vi "Update Item.vi"(8 "error in (no error)":errorcluster, 9 "Tag":string, 10 "Tree Manager in":refnum<class "Tree Manager.lvclass">, 11 "Data Item in":refnum<class "Data Item.lvclass">) -> (0 "error out":errorcluster, 2 "Tree Manager out":refnum<class "Tree Manager.lvclass">, 3 "Data Item out":refnum<class "Data Item.lvclass">)   [LabVIEW 2026, in "VILab.lvlib" / "Data Item.lvclass"]
uses:
  Data Item.lvclass
  Data Item.lvclass/Data Item.ctl
  Tree Manager/Tree Manager.lvclass
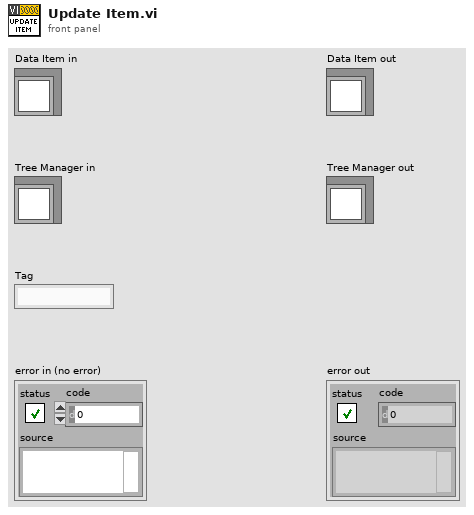
[diagram p1: front panel]
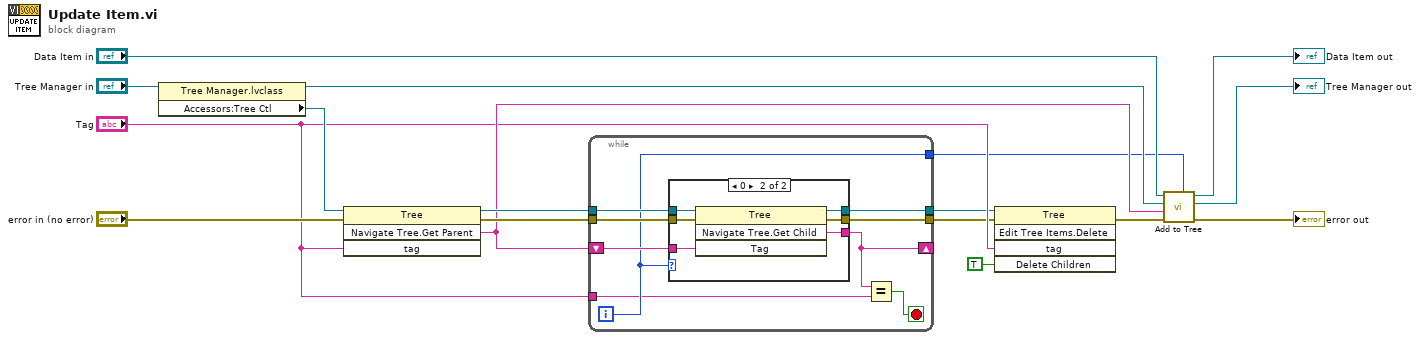
[diagram p0: block diagram]
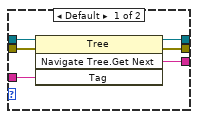
[diagram p2: hidden frame]
diagram:
  n1 = property class="Tree Manager.lvclass"(reference="Tree Manager in") -> (reference out=w16:refnum<class "Tree Manager.lvclass">, "Accessors:Tree Ctl"=w15:refnum<vi>)  [unwired: 1 in, 1 out]
  n2 = invoke class="Tree" method="Navigate Tree.Get Parent"(reference=w15, error in="error in (no error)", "tag"="Tag") -> (reference out=w6:refnum<vi>, error out=w7:errorcluster, "Navigate Tree:Get Parent"=w5:string)  [unwired: 1 in, 1 out]
  n3 = while {
    tunnel: w7 -> [w26]
    tunnel: w6 -> [w25]
    shift-right: [w20] -> _
    shift-left: w5 -> [w24]
    tunnel: [w23] -> w3
    tunnel: "Tag" -> [w21]
    tunnel: [w19] -> w2
    tunnel: [w18] -> w1
    i -> [w23]
    stop <- w22 stop-if-true
    n4 = case shown="0" w23 {
      tunnel: w26 -> [w29 w38]
      tunnel: w25 -> [w32 w37]
      tunnel: w24 -> [w30 w36]
      tunnel: [w31 w35] -> w20
      tunnel: [w28 w34] -> w19
      tunnel: [w27 w33] -> w18
      frame Default {
        n5 = invoke class="Tree" method="Navigate Tree.Get Next"(reference=w32, error in=w29, "Tag"=w30) -> (reference out=w27:refnum<vi>, error out=w28:errorcluster, "Navigate Tree:Get Next Item"=w31:string)  [unwired: 1 in, 1 out]
      }
      frame 0 {
        n6 = invoke class="Tree" method="Navigate Tree.Get Child"(reference=w37, error in=w38, "Tag"=w36) -> (reference out=w33:refnum<vi>, error out=w34:errorcluster, "Navigate Tree:Get Child"=w35:string)  [unwired: 1 in, 1 out]
      }
    }
    n7 = Equal?(x=w20, y=w21) -> (x = y?=w22:bool)
  }
  n8 = invoke on="Delete" class="Tree" method="Edit Tree Items.Delete"(reference=w1, error in=w2, "tag"="Tag", "Delete Children"=TRUE ("Delete Children?")) -> (error out=w8:errorcluster)  [unwired: 1 in, 4 out]
  n9 = call-dynamic "Add to Tree.vi"("Child Position"=w3, "error in (no error)"=w8, "Parent Tag"=w5, "Tree Manager in"=w16, "Data Item in"="Data Item in") -> ("error out"=→"error out":errorcluster, "Tree Manager out"=→"Tree Manager out":refnum<class "Tree Manager.lvclass">, "Data Item out"=→"Data Item out":refnum<class "Data Item.lvclass">)  [unwired: 4 in]
